vi "CreatePrivateEvents.vi"(8 "error in (no error)":errorcluster, 11 "MC":refnum<class "MC.lvclass">) -> (0 "error out":errorcluster, 3 "MC out":refnum<class "MC.lvclass">)   [LabVIEW 2017, in "MC.lvclass"]
doc: "JKI State Machine Objects (SMO) 1.0.2.13\nJKI - JKI\nCopyright (c) 2016, JKI"
uses:
  MC.lvclass
  Typedefs/PrivateEvents--MC.SetWavelength.ctl
  Device/Device.lvclass
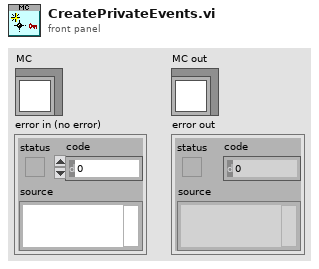
[diagram p1: front panel]
types:
  T1 = typedef "MC.lvclass/PrivateData--Ref.ctl" = refnum<data-value>
  T2 = typedef "MC.lvclass/PrivateEvents--MC.SetWavelength.ctl" = cluster{"Wavelength, nm":dbl}
  T3 = typedef "MC.lvclass/PrivateData--Cluster.ctl" = cluster{"Private Events":T4, "Configuration":T5}
  T4 = typedef "MC.lvclass/PrivateEvents--Cluster.ctl" = cluster{"SetWavelength":refnum<user-event>}
  T5 = typedef "MC.lvclass/Configuration--Cluster.ctl" = cluster{"VISA Resource":string}
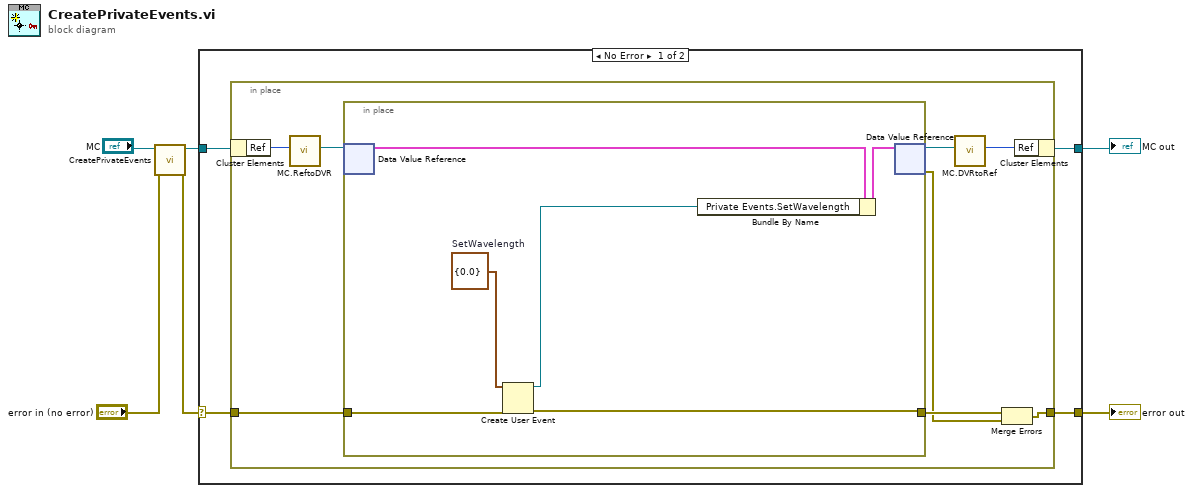
[diagram p0: block diagram]
diagram:
  n1 = call-parent "CreatePrivateEvents.vi"("error in (no error)"="error in (no error)", "SMO"="MC") -> ("error out"=w5:errorcluster, "SMO out"=w6:refnum<class "MC.lvclass">)  [unwired: 8 in]
  n2 = case shown="No Error" w5 {
    selector: w5 -> [w8 w26]
    tunnel: [w7 w26] -> w1
    tunnel: [w9 w25] -> w3
    tunnel: w6 -> [w10 w25]
    frame No Error {
      n3 = in-place {
        in-place-border: w8 -> [w18]
        in-place-border: [w15] -> w7
        n4 = in-place-cluster #1(w10) -> ("Ref"=w14:u32)
        n5 = call "MC.ReftoDVR.vi"("Ref"=w14) -> ("Ref"=w13:T1)  [unwired: 10 in]
        n6 = in-place {
          in-place-border: w18 -> [w23]
          in-place-border: [w21] -> w17
          w20 = T2 {"Wavelength, nm"=0.0}  # SetWavelength
          n7 = in-place-dvr #2(w13) -> (w22:T3)  [unwired: 1 out]
          n8 = Create User Event(user event datatype=w20, error in=w23) -> (user event=w19:refnum<user-event>, error out=w21:errorcluster)
          n9 = Bundle By Name(cluster=w22, "Private Events.SetWavelength"=w19) -> (w24:T3)
          n10 = in-place-dvr #2(w24) -> (w12:T1, w16:errorcluster)
        }
        n11 = call "MC.DVRtoRef.vi"("Ref"=w12) -> ("Ref"=w11:u32)  [unwired: 10 in]
        n12 = Merge Errors(w17, w16) -> (w15:errorcluster)
        n13 = in-place-cluster #1("Ref"=w11) -> (w9:refnum<class "MC.lvclass">)
      }
    }
    frame Error {
    }
  }
  "error out" <- w1
  "MC out" <- w3
